vi "Cmd Set Command Properties (CR).vi"(4 "error in (no error)":errorcluster, 5 "command properties":T1, 7 "command-recordset reference":T2) -> (0 "error out":errorcluster, 3 "command-recordset reference out":T2)   [LabVIEW 2020, in "NI_Database_API.lvlib"]
doc: "Sets properties on the object as determined by the inputs. Wire data to the reference and properties inputs to determine the polymorphic instance to use or manually select the instance."
uses:
  <vilib>/addons/database/NI_Database_API.lvlib
  <vilib>/addons/database/Command-Recordset.llb/Cmd-Rec Object Reference.ctl
  <vilib>/addons/database/Command.llb/Cmd Properties.ctl
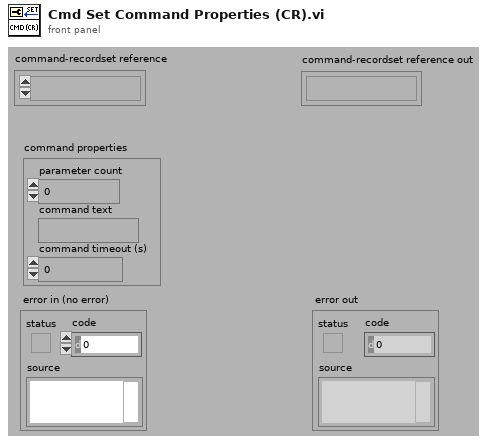
[diagram p1: front panel]
types:
  T1 = typedef "NI_Database_API.lvlib/Cmd Properties.ctl" = cluster{"parameter count":i32, "command text":string, "command timeout (s)":i32}
  T2 = typedef "NI_Database_API.lvlib/Cmd-Rec Object Reference.ctl" = refnum<k1>
  T3 = typedef "NI_Database_API.lvlib/Cmd-Rec Data Members.ctl" = cluster{"recordset reference":T4, "command reference":T5}
  T4 = typedef "NI_Database_API.lvlib/Rec ObjectReference.ctl" = refnum<k1>
  T5 = typedef "NI_Database_API.lvlib/Cmd ObjectReference.ctl" = refnum<k1>
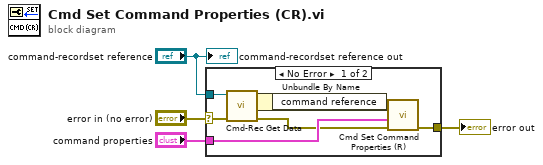
[diagram p0: block diagram]
diagram:
  n1 = case shown="No Error" "error in (no error)" {
    selector: "error in (no error)" -> [w5 w12]
    tunnel: [w11 w12] -> w4
    tunnel: "command properties" -> [w10 _]
    tunnel: "command-recordset reference" -> [w8 _]
    frame No Error {
      n2 = call <vilib>:"Cmd-Rec Get Data.vi"("error in (no error)"=w5, "command-recordset reference"=w8) -> ("error out"=w6:errorcluster, "data"=w9:T3)  [unwired: 2 in, 2 out]
      n3 = Unbundle By Name(w9) -> ("command reference"=w7:T5)
      n4 = call <vilib>:"Cmd Set Command Properties (R).vi"("error in (no error)"=w6, "command properties"=w10, "command reference"=w7) -> ("error out"=w11:errorcluster)  [unwired: 3 in, 1 out]
    }
    frame Error {
    }
  }
  "error out" <- w4
  "command-recordset reference out" <- "command-recordset reference"
